vi "SPAN Table.vi"(6 "Sprachliste":string[][](array[string]), 8 "Fehler (Eingang, kein Fehler)":errorcluster, 11 "SpanComponentInfos-Cluster":T1) -> (0 "Fehler (Ausgang)":errorcluster, 3 "SpanTable Info Array":string[][](array[string]))   [LabVIEW 2020, in "Linearisierung v2.lvlib" / "Protokoll.lvlib"]
uses:
  Protokoll.lvlib
  SpanEinstellungen/SpanComponentInfos-Cluster.ctl
  SpanEinstellungen/ComponentInfos.ctl
  Visualisierungs Elemente/String - Ausgabefeld.ctl
  Visualisierungs Elemente/String - Eingabefeld.ctl
  Gasteiler/HovaCAL_Interface/Kommunikation/Aktion FGV HovaCAL Interface Autolin.ctl
  Gasteiler/Aktionen FGV Gasteiler Daten.ctl
  GasteilerType.ctl
  SpanEinstellungen/SpanEinstellungen.lvlib
  Sprachverwaltung/Sprachverwaltung.lvlib
  Gasteiler/HovaCAL_Interface/Kommunikation/Kommunikation.lvlib
  Gasteiler/Gasteiler.lvlib
  Linearisierung v2.lvlib
  Gasteiler/HovaCAL_Interface/Helper/Helper.lvlib
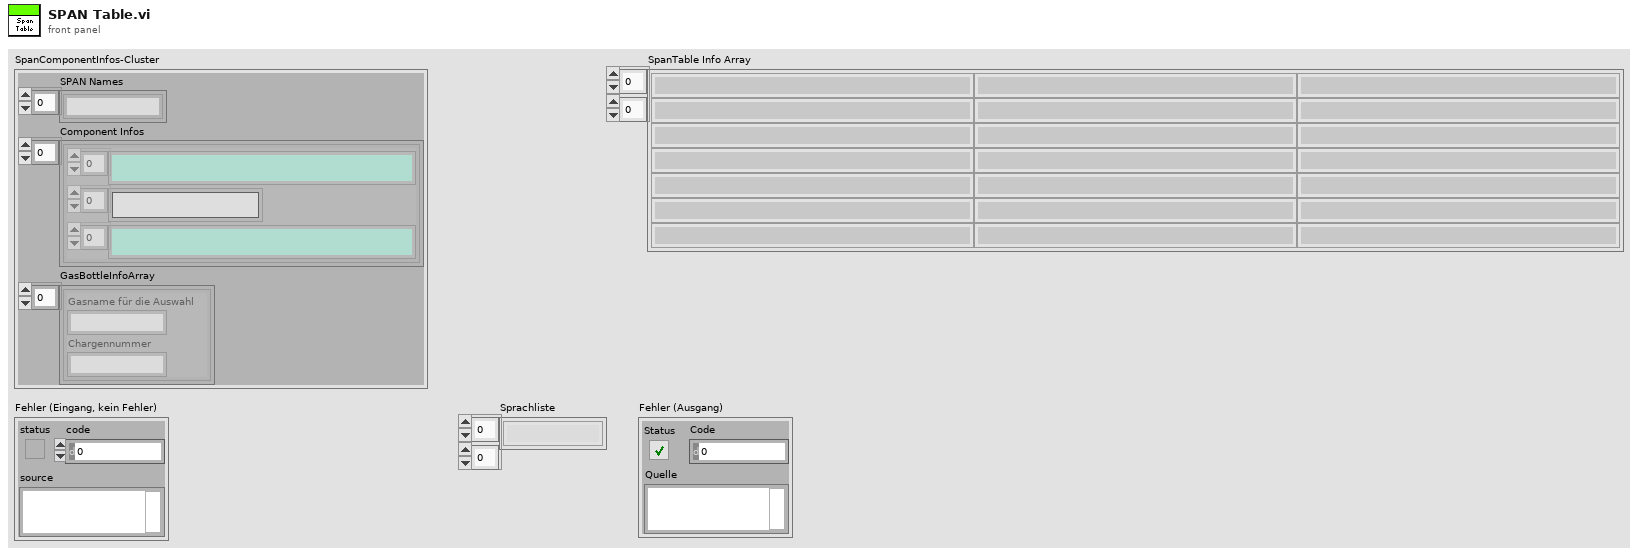
[diagram p1: front panel]
types:
  T1 = typedef "Linearisierung v2.lvlib/SpanEinstellungen.lvlib/SpanComponentInfos-Cluster.ctl" = cluster{"SPAN Names":string[], "Component Infos":T2[], "GasBottleInfoArray":cluster{"Gasname für die Auswahl":string, "Chargennummer":string}[]}
  T2 = typedef "Linearisierung v2.lvlib/SpanEinstellungen.lvlib/ComponentInfos.ctl" = cluster{T3[], T4[], T3[]}
  T3 = typedef "String - Ausgabefeld.ctl" = string
  T4 = typedef "String - Eingabefeld.ctl" = string
  T5 = typedef "Linearisierung v2.lvlib/GasteilerType.ctl" = u16
  T6 = typedef "Linearisierung v2.lvlib/Gasteiler.lvlib/Aktionen FGV Gasteiler Daten.ctl" = enum16{"lesen", "Gasteiler Daten", "Seriellen Param.", "MB-Endwert", "laden", "speichern", "Anforderung", "TCP", "Aufzeichnung Start"}
  T7 = typedef "Linearisierung v2.lvlib/Gasteiler.lvlib/HovaCAL_Interface.lvlib/Kommunikation.lvlib/Aktion FGV HovaCAL Interface Autolin.ctl" = enum16{"lesen", "schreiben", "MFC Komponente fix setzen", "init"}
  T8 = cluster{"Gasname für die Auswahl":string, "Chargennummer":string}[]
  T9 = typedef "Linearisierung v2.lvlib/Gasteiler.lvlib/Gasteiler Daten.ctl" = cluster{"Gasteiler":T4, "Gasteiler Stufen":T10, "Gasteiler Type":T5, "Konfig Gasteiler":T11, "Gasteiler Span Eingänge":u16}
  T10 = typedef "Linearisierung v2.lvlib/Gasteiler.lvlib/Gasteiler Stufen.ctl" = u16
  T11 = typedef "System Einstellungen V2.lvlib/Gasteiler Auswahl.ctl" = u16
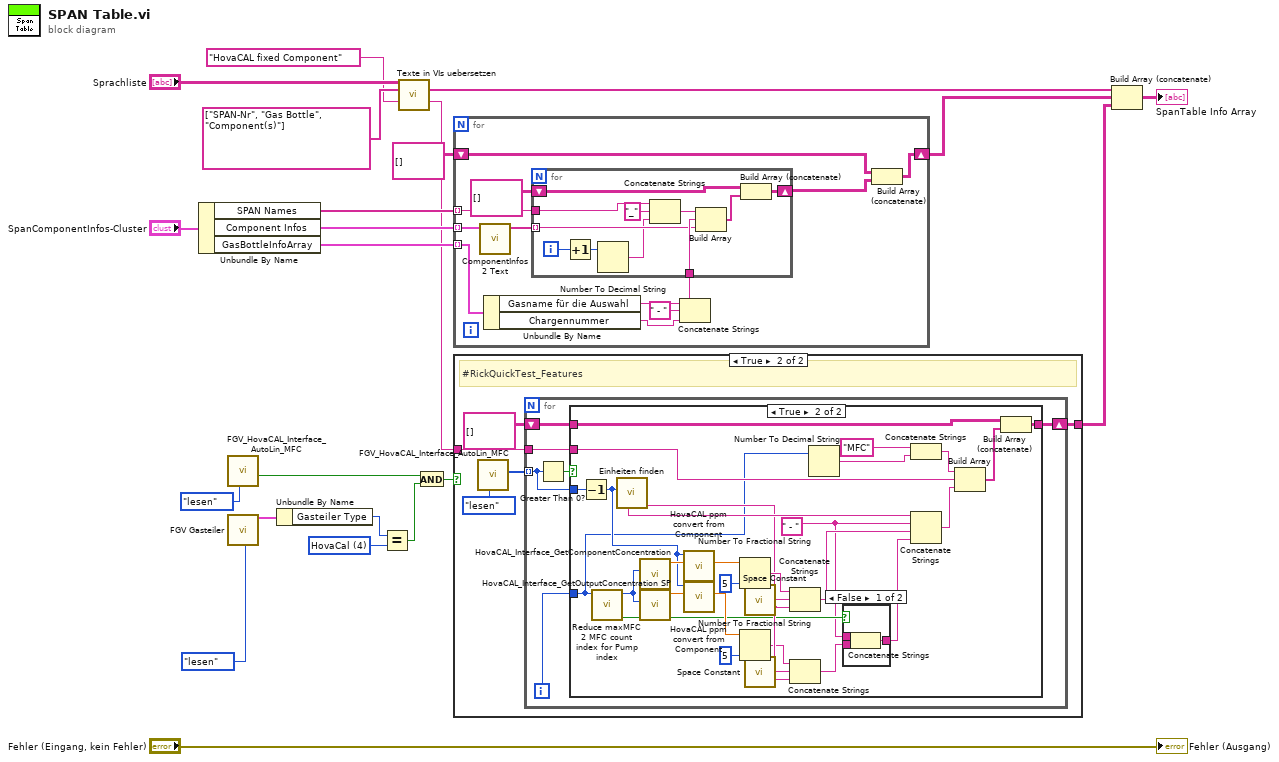
[diagram p0: block diagram]
diagram:
  w9 = T5 4 items=["LNI", "Analog-Display", "AVL GDU", "Horiba GDC", "HovaCal", "Horiba SGD 710C"] ("y")
  n1 = Unbundle By Name("SpanComponentInfos-Cluster") -> ("SPAN Names"=w21:string[], "Component Infos"=w20:T2[], "GasBottleInfoArray"=w19:T8)
  n2 = call "FGV_HovaCAL_Interface_AutoLin_MFC.vi"("Aktion"=Aktion_FGV_HovaCAL_Interface_Autolin."lesen") -> ("fix conf"=w5:bool)  [unwired: 7 in, 3 out]
  n3 = call "FGV Gasteiler.vi"("Aktionen"=Aktionen_FGV_Gasteiler_Daten."lesen") -> ("Gasteiler Daten"=w11:T9)  [unwired: 11 in, 7 out]
  n4 = Unbundle By Name(w11) -> ("Gasteiler Type"=w10:T5)
  n5 = Equal?(x=w10, y=w9) -> (x = y?=w6:bool)
  n6 = call "Texte in VIs uebersetzen.vi"("Sprachliste"="Sprachliste", "String-Array zum Übersetzen"=string[] ["SPAN-Nr", "Gas Bottle", "Component(s)"], "String zum Übersetzen"=T3 "HovaCAL fixed Component" ("String")) -> ("String-Array zum Übersetzen"=w14:string[], "String zum Übersetzen"=w2:string)  [unwired: 8 in, 3 out]
  n7 = And(x=w5, y=w6) -> (x .and. y?=w4:bool)
  n8 = for {
    tunnel: w21 -> [w33] mode=indexing
    tunnel: w20 -> [w34] mode=indexing
    tunnel: w19 -> [w32] mode=indexing
    shift-right: [w26] -> w13
    shift-left: string[][] [] -> [w25]
    n9 = call "ComponentInfos 2 Text.vi"("Component Infos"=w34) -> ("Component Text Array"=w24:T3[])  [unwired: 10 in]
    n10 = Unbundle By Name(w32) -> ("Gasname für die Auswahl"=w31:string, "Chargennummer"=w29:string)
    n11 = Concatenate Strings(w31, " - " ("String"), w29) -> (w28:string)
    n12 = for {
      tunnel: w33 -> [w45]
      tunnel: w28 -> [w44]
      tunnel: w24 -> [w43] mode=indexing
      shift-right: [w42] -> w27
      shift-left: T3[][] [] -> [w36]
      i -> [w40]
      n13 = Increment(x=w40) -> (x+1=w39:i32)
      n14 = Number To Decimal String(number=w39) -> (decimal integer string=w37:string)  [unwired: 1 in]
      n15 = Concatenate Strings(w45, "_" ("String"), w37) -> (w41:string)
      n16 = Build Array(w41, w44, w43) -> (w35:T3[])
      n17 = Build Array (concatenate)(w36, w35) -> (w42:T3[][])
    }
    n18 = Build Array (concatenate)(w25, w27) -> (w26:T3[][])
  }
  n19 = case shown="True" w4 {
    tunnel: w2 -> [_ w48]
    tunnel: [_ w46] -> w1
    frame False {
    }
    frame True {
      # "#RickQuickTest_Features"
      n20 = call "FGV_HovaCAL_Interface_AutoLin_MFC.vi"("Aktion"=Aktion_FGV_HovaCAL_Interface_Autolin."lesen") -> ("MFV Komponente fix out"=w49:u16[])  [unwired: 7 in, 3 out]
      n21 = for {
        tunnel: w49 -> [w55] mode=indexing
        tunnel: w48 -> [w53]
        shift-right: [w52] -> w46
        shift-left: string[][] [] -> [w51]
        i -> [w54]
        n22 = Greater Than 0?(x=w55) -> (x > 0?=w56:bool)
        n23 = case shown="True" w56 {
          tunnel: w55 -> [_ w86]
          tunnel: w54 -> [_ w62]
          tunnel: w53 -> [_ w65]
          tunnel: [w57 w59] -> w52
          tunnel: w51 -> [w57 w58]
          frame False {
          }
          frame True {
            w69 = " - " ("String")
            n24 = Decrement(x=w86) -> (x-1=w82:u16)
            n25 = call "Reduce maxMFC 2 MFC count index for Pump index.vi"("MFC idx"=w62) -> ("Pump"=w70:bool, "AutoLin MFC"=w85:i32)  [unwired: 8 in, 1 out]
            n26 = call "Einheiten finden.vi"("Komponente"=w82) -> ("Einheit in String"=w73:string, "Komponenten Name"=w80:T3)  [unwired: 6 in, 3 out]
            n27 = call "HovaCAL_Interface_GetComponentConcentration.vi"("AutoLin MFV Index"=w85) -> ("Konzentration"=w84:dbl)  [unwired: 8 in, 2 out]
            n28 = call "HovaCAL_Interface_GetOutputConcentration SP.vi"("AutoLin MFC Index"=w85) -> ("Konzentration"=w83:dbl)  [unwired: 8 in, 2 out]
            n29 = call "HovaCAL ppm convert from Component.vi"("Konzentration"=w84, "Gasnummer"=w82) -> ("Konzentration in %"=w79:dbl)  [unwired: 5 in, 4 out]
            n30 = call "HovaCAL ppm convert from Component.vi"("Konzentration"=w83, "Gasnummer"=w82) -> ("Konzentration in %"=w72:dbl)  [unwired: 5 in, 4 out]
            n31 = Number To Fractional String(number=w79, precision (6)=i16 5 ("Genauigkeit (6)")) -> (F-format string=w77:string)  [unwired: 2 in]
            n32 = Number To Fractional String(number=w72, precision (6)=i16 5 ("Genauigkeit (6)")) -> (F-format string=w71:string)  [unwired: 2 in]
            n33 = call <vilib>:"Space Constant.vi"() -> ("String"=w78:string)
            n34 = call <vilib>:"Space Constant.vi"() -> ("String"=w75:string)
            n35 = Concatenate Strings(w77, w78, w73) -> (w76:string)
            n36 = Concatenate Strings(w71, w75, w73) -> (w68:string)
            n37 = Number To Decimal String(number=w62) -> (decimal integer string=w61:string)  [unwired: 1 in]
            n38 = case shown="False" w70 {
              tunnel: w68 -> [w89 _]
              tunnel: w69 -> [w88 _]
              tunnel: [w87 _] -> w67
              frame False {
                n39 = Concatenate Strings(w88, w89) -> (w87:string)
              }
              frame True {
              }
            }
            n40 = Concatenate Strings("MFC", w61) -> (w64:string)
            n41 = Concatenate Strings(w80, w69, w76, w67) -> (w66:string)
            n42 = Build Array(w64, w65, w66) -> (w60:string[])
            n43 = Build Array (concatenate)(w58, w60) -> (w59:string[][])
          }
        }
      }
    }
  }
  n44 = Build Array (concatenate)(w14, w13, w1) -> (→"SpanTable Info Array":T3[][])
  "Fehler (Ausgang)" <- "Fehler (Eingang, kein Fehler)"
